vi "Initialize.vi"(8 "error in (no error)":errorcluster, 9 "Reset (yes)":bool=TRUE, 10 "ID Query (yes)":bool=TRUE, 11 "VISA resource name":refnum<visa-resource-name>) -> (0 "error out":errorcluster, 3 "VISA resource name out":refnum<visa-resource-name>)   [LabVIEW 2016, in "Agilent 4263X.lvlib"]
doc: "Passes the addressing information in the instrument descriptor control to the VISA Open VI and returns the instrument ID to be used with other driver VIs."
uses:
  <instrlib>/Agilent 4263X/Agilent 4263X.lvlib
panel:
  # "yes\nno"
  # "yes\nno"
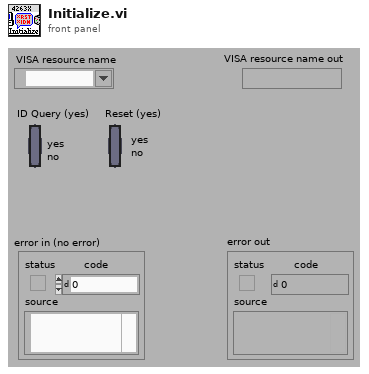
[diagram p1: front panel]
types:
  T1 = cluster{"status":bool, "code":i32, "VI name":string}
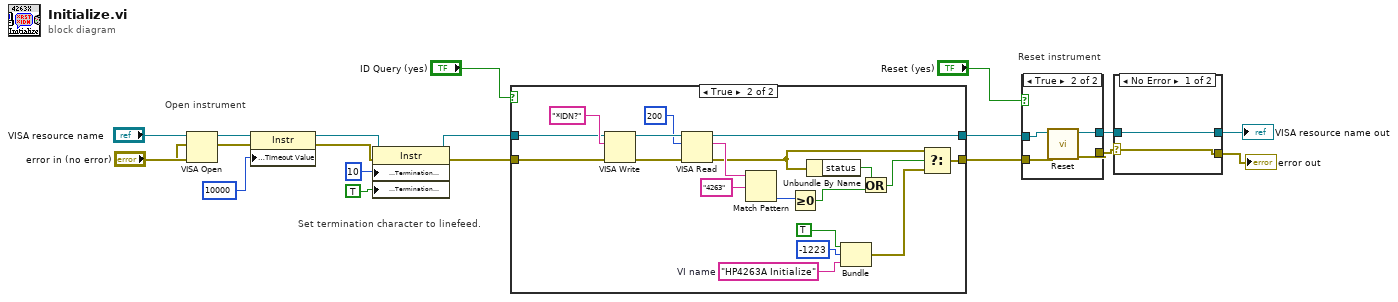
[diagram p0: block diagram]
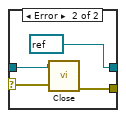
[diagram p2: hidden frame]
diagram:
  # "Reset instrument"
  # "Set termination character to linefeed."
  # "Open instrument"
  n1 = VISA Open(error in (no error)="error in (no error)", VISA resource name="VISA resource name") -> (VISA resource name=w16:refnum<visa-resource-name>, error out=w15:errorcluster)  [unwired: 3 in]
  n2 = property on="Property Node" class="Instr"(reference=w16, error in=w15, "General Settings:Timeout Value"=u32 10000 ("Tmo Value")) -> (reference out=w9:refnum<visa-resource-name>, error out=w8:errorcluster)
  n3 = property on="Property Node" class="Instr"(reference=w9, error in=w8, "Message Based Settings:Termination Character"=10, "Message Based Settings:Termination Character Enable"=TRUE) -> (reference out=w10:refnum<visa-resource-name>, error out=w7:errorcluster)
  n4 = case shown="True" "ID Query (yes)" {
    tunnel: w7 -> [w20 w36]
    tunnel: [w21 w34] -> w6
    tunnel: w10 -> [w21 w37]
    tunnel: [w20 w22] -> w5
    frame False {
    }
    frame True {
      w23 = "HP4263A Initialize"  # VI name
      n5 = VISA Write(VISA resource name=w37, write buffer="*IDN?", error in (no error)=w36) -> (VISA resource name out=w31:refnum<visa-resource-name>, error out=w35:errorcluster)  [unwired: 1 out]
      n6 = VISA Read(VISA resource name=w31, byte count=200, error in (no error)=w35) -> (VISA resource name out=w34:refnum<visa-resource-name>, read buffer=w32:string, error out=w25:errorcluster)  [unwired: 1 out]
      n7 = Match Pattern(string=w32, regular expression="4263") -> (offset past match=w26:i32)  [unwired: 1 in, 3 out]
      n8 = Greater Or Equal To 0?(x=w26) -> (x >= 0?=w27:bool)
      n9 = Unbundle By Name(w25) -> ("status"=w28:bool)
      n10 = Bundle(TRUE, -1223, "VI name"=w23) -> (w29:cluster{bool, i32, "VI name":string})  [unwired: 1 in]
      n11 = Or(x=w28, y=w27) -> (x .or. y?=w24:bool)
      n12 = Select(t=w25, s=w24, f=w29) -> (s? t:f=w22:T1)
    }
  }
  n13 = case shown="True" "Reset (yes)" {
    tunnel: [w42 w44] -> w4
    tunnel: w6 -> [w41 w46]
    tunnel: w5 -> [w42 w45]
    tunnel: [w41 w43] -> w3
    frame False {
    }
    frame True {
      n14 = call <instrlib>:"Reset.vi"("error in (no error)"=w45, "VISA resource name"=w46) -> ("error out"=w44:errorcluster, "VISA resource name out"=w43:refnum<visa-resource-name>)  [unwired: 8 in]
    }
  }
  n15 = case shown="No Error" w4 {
    selector: w4 -> [w47 w51]
    tunnel: w3 -> [w48 w52]
    tunnel: [w47 w50] -> w2
    tunnel: [w48 refnum<visa-resource-name> refnum ("VISA resource name out")] -> w1
    frame No Error {
    }
    frame Error {
      n16 = call <instrlib>:"Close.vi"("error in (no error)"=w51, "VISA resource name"=w52) -> ("error out"=w50:errorcluster)  [unwired: 9 in]
    }
  }
  "error out" <- w2
  "VISA resource name out" <- w1
